vi "page3.vi"() -> ()   [LabVIEW 2013]
uses:
  App Buttons.ctl
panel:
  in  "OK Button 11":T1
  in  "OK Button 10":T1
  in  "OK Button 9":T1
  in  "OK Button 8":T1
  in  "OK Button 7":T1
  in  "OK Button 6":T1
  in  "OK Button 5":T1
  in  "OK Button 4":T1
  in  "OK Button 3":T1
  in  "OK Button 2":T1
  in  "stop":bool
  out "Boolean":bool
  # "Page 3"
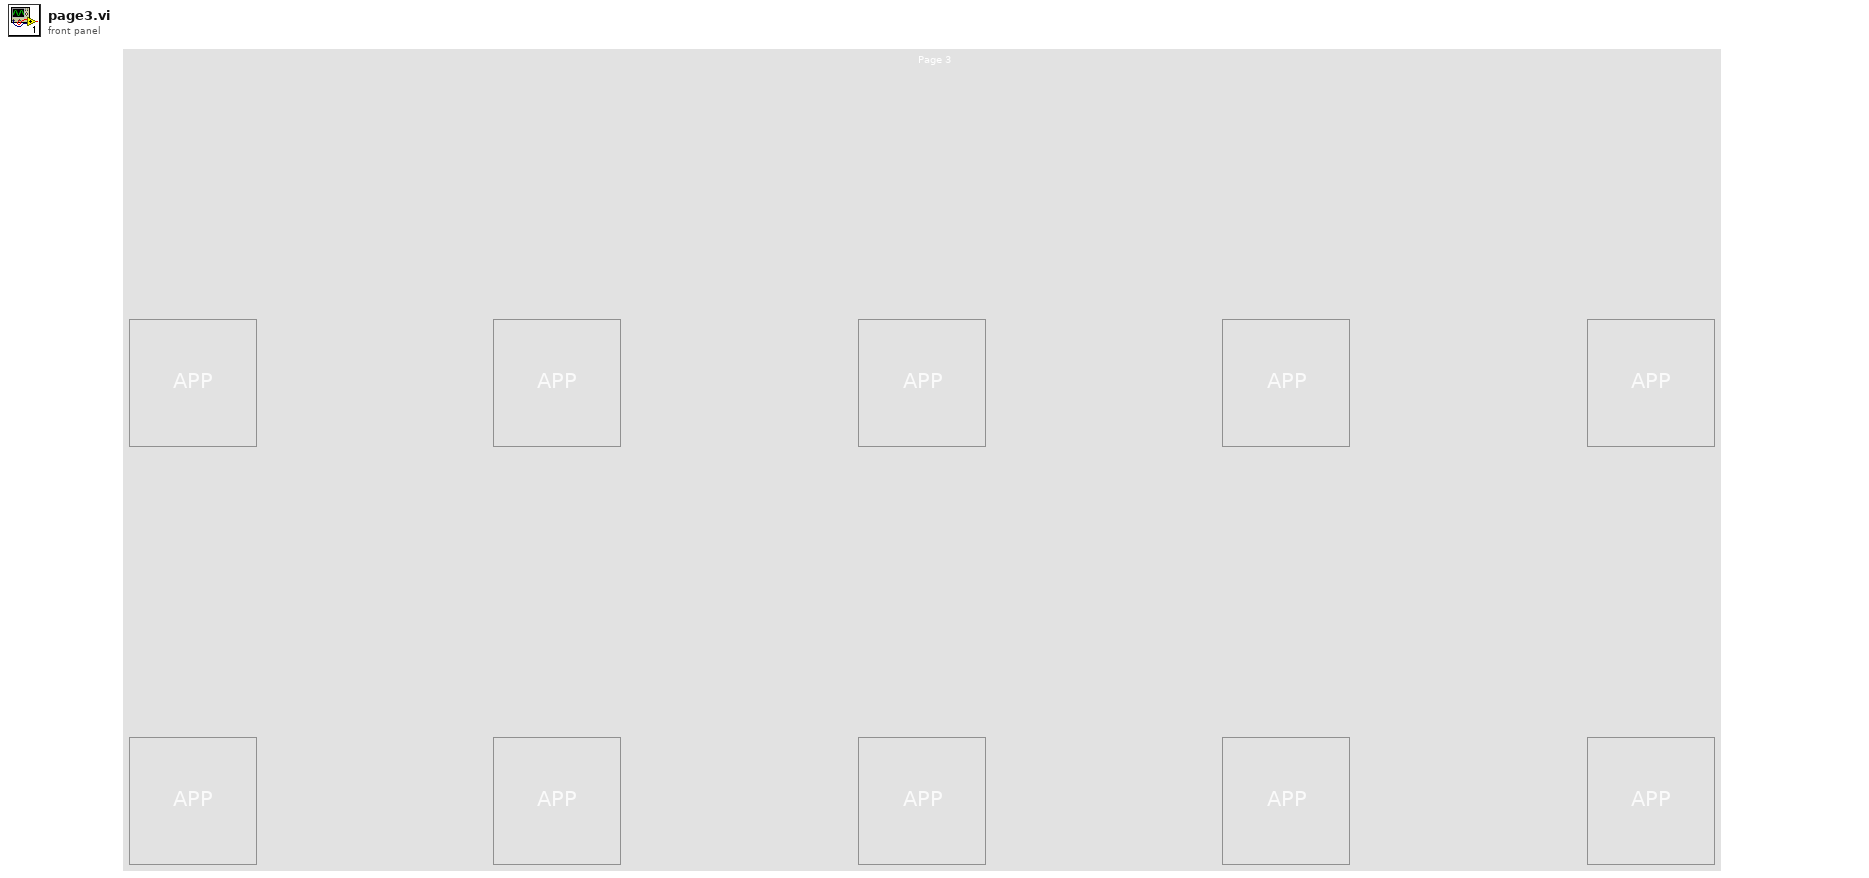
[diagram p1: front panel]
types:
  T1 = typedef "App Buttons.ctl" = bool
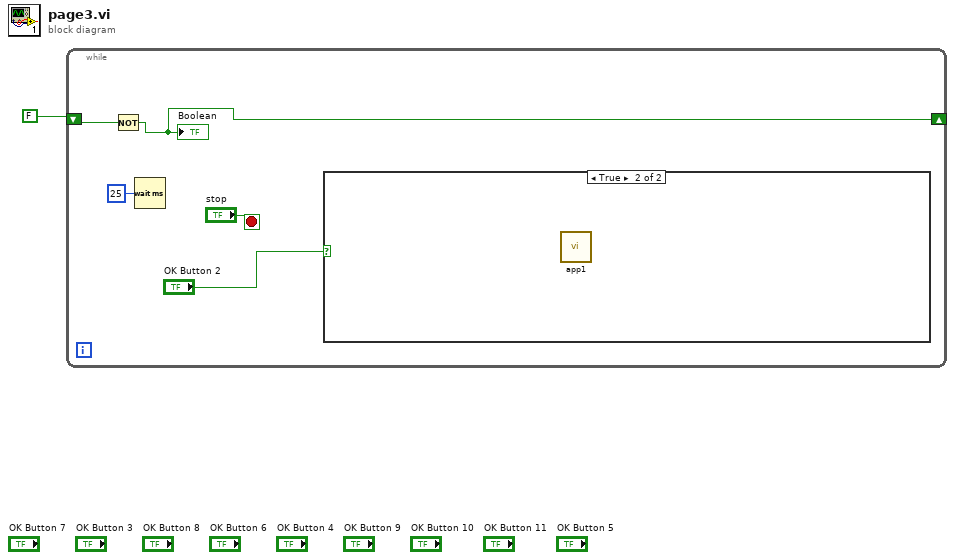
[diagram p0: block diagram]
diagram:
  n1 = while {
    shift-right: [w4] -> _
    shift-left: FALSE ("Boolean") -> [w5]
    stop <- "stop" stop-if-true
    n2 = Not(x=w5) -> (.not. x?=w4:bool)
    "Boolean" <- w4
    n3 = Wait (ms)(milliseconds to wait=u32 25) -> ()  [unwired: 1 out]
    n4 = case shown="True" "OK Button 2" {
      frame False {
      }
      frame True {
        n5 = call "app1.vi"() -> ()  [unwired: 12 in]
      }
    }
  }
